vi "FA25_FW_pendulum_L3_4_0.vi"() -> ()   [LabVIEW 2025]
uses:
  <vilib>/Analysis/3filter.llb/Filter Passband Type.ctl
  Lab 3/FA25_pend_Lab3_4/SADI_Pendulum_lib/pendulumApp.lvlib
  <vilib>/ptbypt/NI_PtbyPt.lvlib
  <vilib>/Analysis/NI_AALBase.lvlib
panel:
  out "command":dbl
  in  "Tab Control":T1(tab)=enum."Plant and Controller"
  out "Firmware Version":sgl=1.002
  out "Software Version":dbl=1.104 format="%_6g"
  out "Number of SADI":i32=1
  out "reset":i32
  out "SADI Connect":i32
  out "P query":i32
  out "P start":i32
  in  "Desired DAQ Loop \nTime (ms)":dbl=0.2
  out "Actual DAQ Loop \nTime (ms)":dbl=0.20860000000084256 format="%#_7g"
  out "Elapsed \nTime (s) daq loop":dbl=15.046546899999953
  out "Txlat_ms":dbl=1.778
  out "min Txlat":dbl=0.682 format="%0.6f"
  out "max TXlat":dbl=4.932 format="%0.6f"
  out "std dev TXlat":dbl=0.7050052541669608 format="%0.6f"
  out "mean  TXlat":dbl=1.2022235999999924 format="%0.6f"
  out "Tx latency, ms":T2(graph)={"X Values"=[0.70325, 0.74575, 0.7882500000000001, 0.8307500000000001, 0.8732500000000001, 0.9157500000000001, 0.95825, 1.00075, 1.04325, 1.0857500000000002, 1.1282500000000002, 1.1707500000000002, 1.2132500000000002, 1.2557500000000001, 1.2982500000000001, 1.34075, 1.38325, 1.42575, 1.46825, 1.51075, 1.55325, 1.59575, 1.63825, 1.68075, 1.72325, 1.76575, 1.8082500000000004, 1.8507500000000003, 1.8932500000000003, 1.9357500000000003, 1.9782500000000003, 2.02075, 2.06325, 2.10575, 2.14825, 2.19075, 2.23325, 2.27575, 2.31825, 2.36075, 2.40325, 2.44575, 2.48825, 2.53075, 2.57325, 2.61575, 2.65825, 2.7007499999999998, 2.7432499999999997, 2.7857499999999997, 2.8282499999999997, 2.8707499999999997, 2.9132499999999997, 2.95575, 2.99825, 3.04075, 3.08325, 3.12575, 3.16825, 3.21075, 3.25325, 3.29575, 3.33825, 3.38075, 3.42325, 3.46575, 3.50825, 3.55075, 3.59325, 3.63575, 3.67825, 3.72075, 3.7632499999999998, 3.8057499999999997, 3.84825, 3.89075, 3.93325, 3.97575, 4.01825, 4.0607500000000005, 4.10325, 4.1457500000000005, 4.18825, 4.2307500000000005, 4.27325, 4.31575, 4.35825, 4.40075, 4.44325, 4.48575, 4.52825, 4.57075, 4.61325, 4.65575, 4.698250000000001, 4.74075, 4.783250000000001, 4.82575, 4.868250000000001, 4.91075], "Histogram: h(x)"=[155, 338, 552, 840, 858, 795, 153, 0, 0, 0, 0, 0, 0, 0, 0, 0, 0, 0, 0, 0, 0, 0, 0, 5, 49, 156, 220, 199, 196, 149, 0, 0, 0, 0, 0, 0, 0, 0, 0, 0, 0, 0, 0, 0, 0, 0, 0, 17, 26, 34, 37, 44, 58, 6, 0, 0, 0, 0, 0, 0, 0, 0, 0, 0, 0, 0, 0, 0, 0, 0, 0, 5, 5, 19, 5, 41, 7, 0, 0, 0, 0, 0, 0, 0, 0, 0, 0, 0, 0, 0, 0, 0, 0, 0, 0, 4, 0, 3, 0, 24]}
  out "ENC VEL":dbl=0.5175486320891765
  out "Pend Rot Error":dbl
  out "Pend Rot Filt":dbl=nan format="%0.2f"
  out "Pendulum velocity":dbl=3.5305560095629e-285
  out "Platen velocity":dbl=0.01738392532814515
  out "Command":dbl=-14.479572053947942
  out "desired\nposition":dbl=-14.790379679306856
  out "Platen Rot Error":dbl format="%0.2f"
  in  "Frequency":dbl=0.5
  in  "Amplitude":dbl=100.0
  in  "Turn On Command":dbl=40.0
  in  "Stop":bool=TRUE
  in  "Desired Loop \nTime (ms)":dbl=1.0
  out "Actual Loop Time (ms)":dbl=1.0000979999995252
  out "Elapsed Time (s)":dbl=15.048252700000035
  out "Segments Saved":u32
  in  "Save Data?":bool
  out "ENC POS":i32=-761
  out "Pendulum ENC":i32
  in  "Sine/Square":bool=TRUE
  in  "Enable Motor":bool=TRUE
  in  "Output Units":enum16{"Degrees", "Radians"}(ring)
  in  "Couts/rev":dbl=3704.0
  in  "Zero":bool
  out "Platen Rotation":dbl=-73.96328293736501
  out "Command Graph":T3(graph)={"Desired Rotation/Command"=-14.479572053947942, -14.479572053947942, 0.0, 0.0}
  out "Desired vs Actual Platen Angle Graph":cluster{"sine wave":dbl, "Filtered x":dbl}(graph)={"sine wave"=-14.479572053947942, "Filtered x"=-73.96328293736501}
  out "Pendulum Rotation Graph":cluster{dbl, dbl}(graph)={nan, 0.0}
  in  "n-int":i32=100
  in  "n-diff":i32=5
  in  "Sampling freq: fs":dbl=1000.0
  in  "Cutoff freq: fl":dbl=10.0 format="%0.3f"
  in  "initialize":bool
  out "PendEncValMax":u16=3687
  out "PendEncValMin":u16=3178
  in  "Pendulum Zero":bool
  out "Pend Rotation":dbl=1440.0 format="%0.2f"
  in  "k1":dbl
  in  "k2":dbl
  in  "k3":dbl
  in  "k4":dbl
  out "u":dbl
  in  "k5":dbl
  out "Read Call Error Out":u16(ring)=32768 items=["SADI_RESET (FT_OK)"=0, "FT_INVALID_HANDLE"=1, "FT_DEVICE_NOT_FOUND"=2, "FT_DEVICE_NOT_OPENED"=3, "FT_IO_ERROR"=4, "FT_INSUFFICIENT_RESOURCES"=5, "FT_OTHER_ERROR"=18, "FT_NOT_SUPPORTED"=17, "DATA_RECEIVED"=32768, "NO_DATA_AVAIL"=32769, "NO_SADI"=32770]
  out "SADI State":T4(ring)=enum."Close"
  # "Platen Rotation & Velocity"
  # "Signal Generator"
  # "Butterworth Filter Settings"
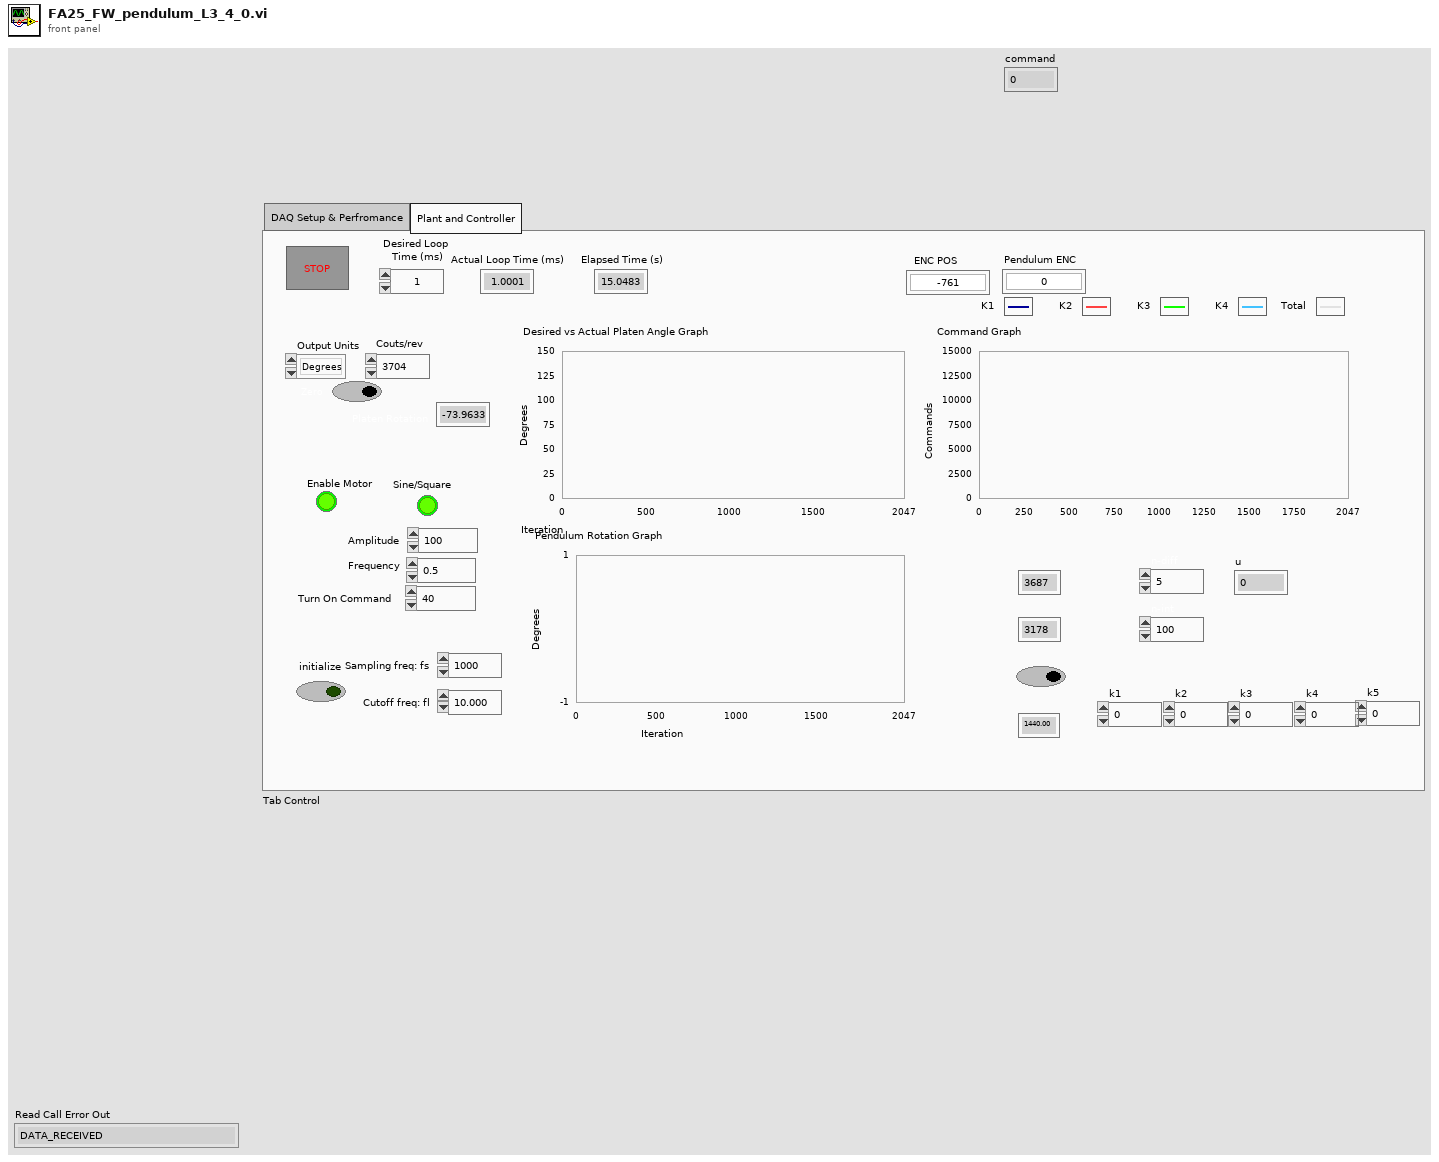
[diagram p1: front panel]
types:
  T1 = enum32{"DAQ Setup & Perfromance", "Plant and Controller"}
  T2 = cluster{"X Values":dbl[], "Histogram: h(x)":i32[]}
  T3 = cluster{"Desired Rotation/Command":dbl, dbl, dbl, dbl}
  T4 = enum32{"SADI_check", "Connect_boot", "Check_SW_FW", "Pend_Start", "Run", "Stop", "Store", "Close"}
  T5 = typedef "NI_AALBase.lvlib/Filter Passband Type.ctl" = enum32{"Lowpass", "Highpass", "Bandpass", "Bandstop"}
  T6 = cluster{"desired\nposition":dbl, "Platen Rotation":dbl}
  T7 = cluster{"desired\nposition":dbl, "Command":dbl, dbl, dbl}
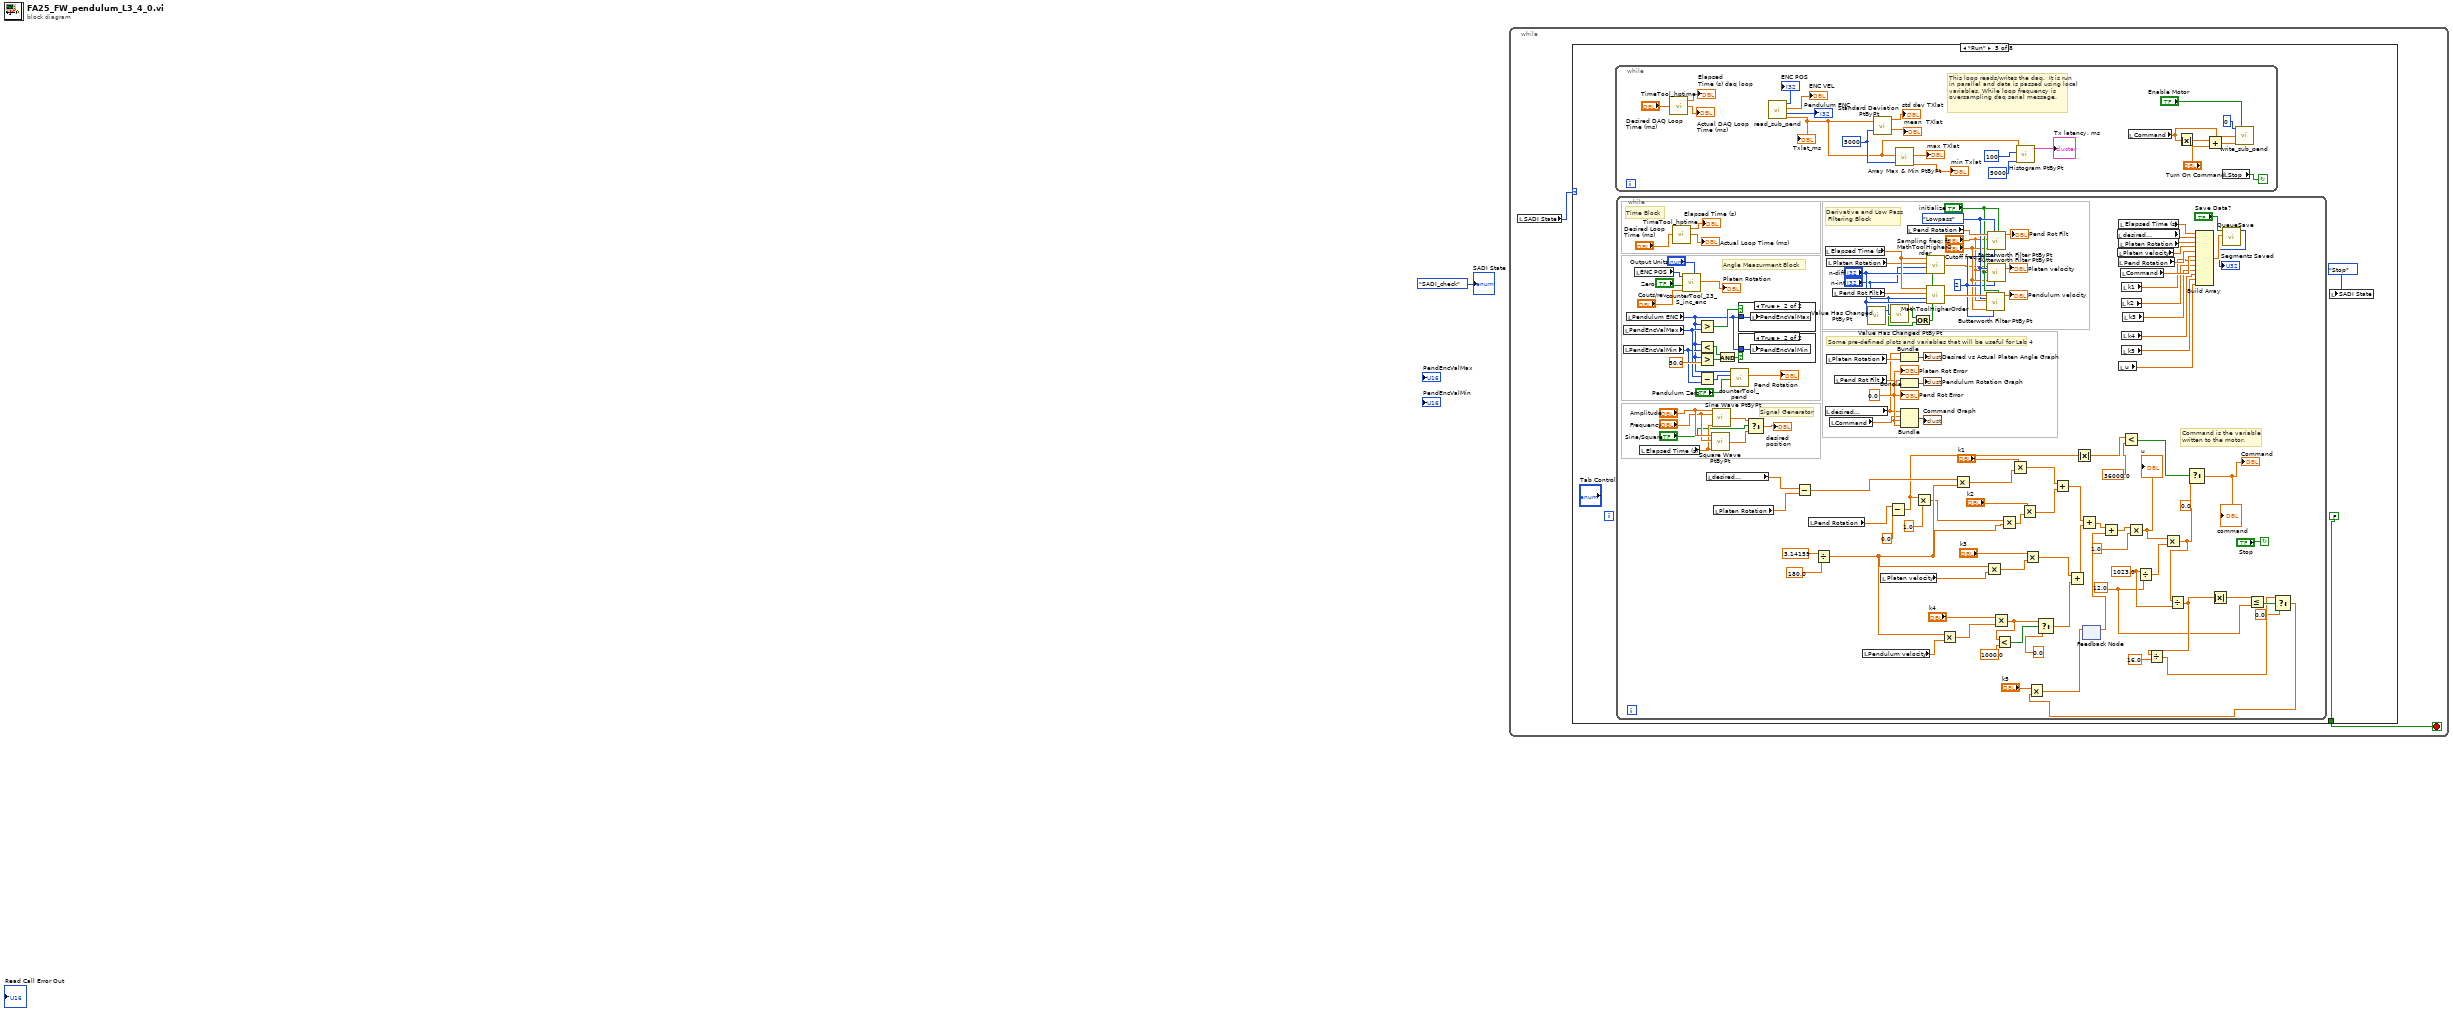
[diagram p0: block diagram]
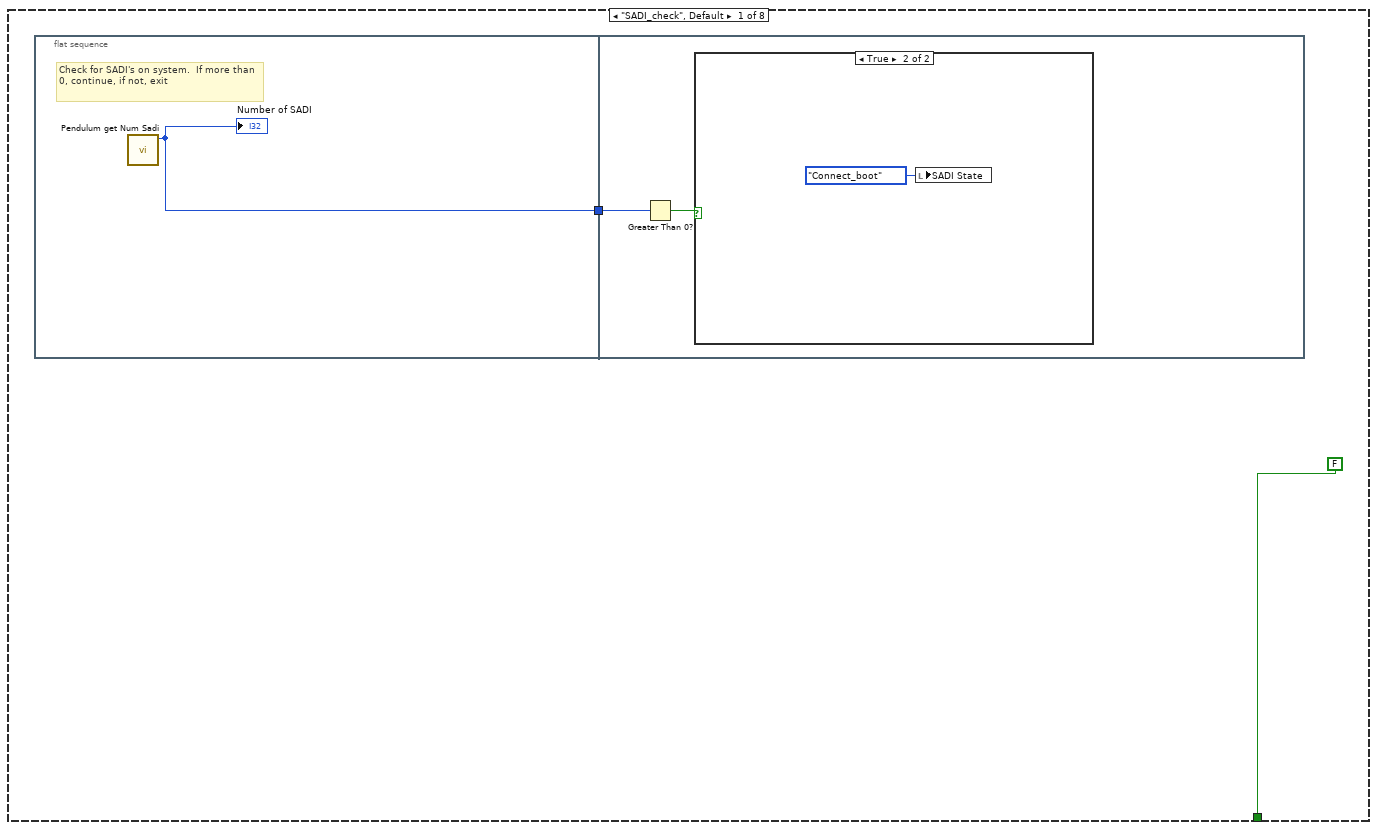
[diagram p2: hidden frame]
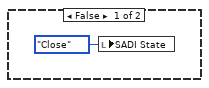
[diagram p3: hidden frame]
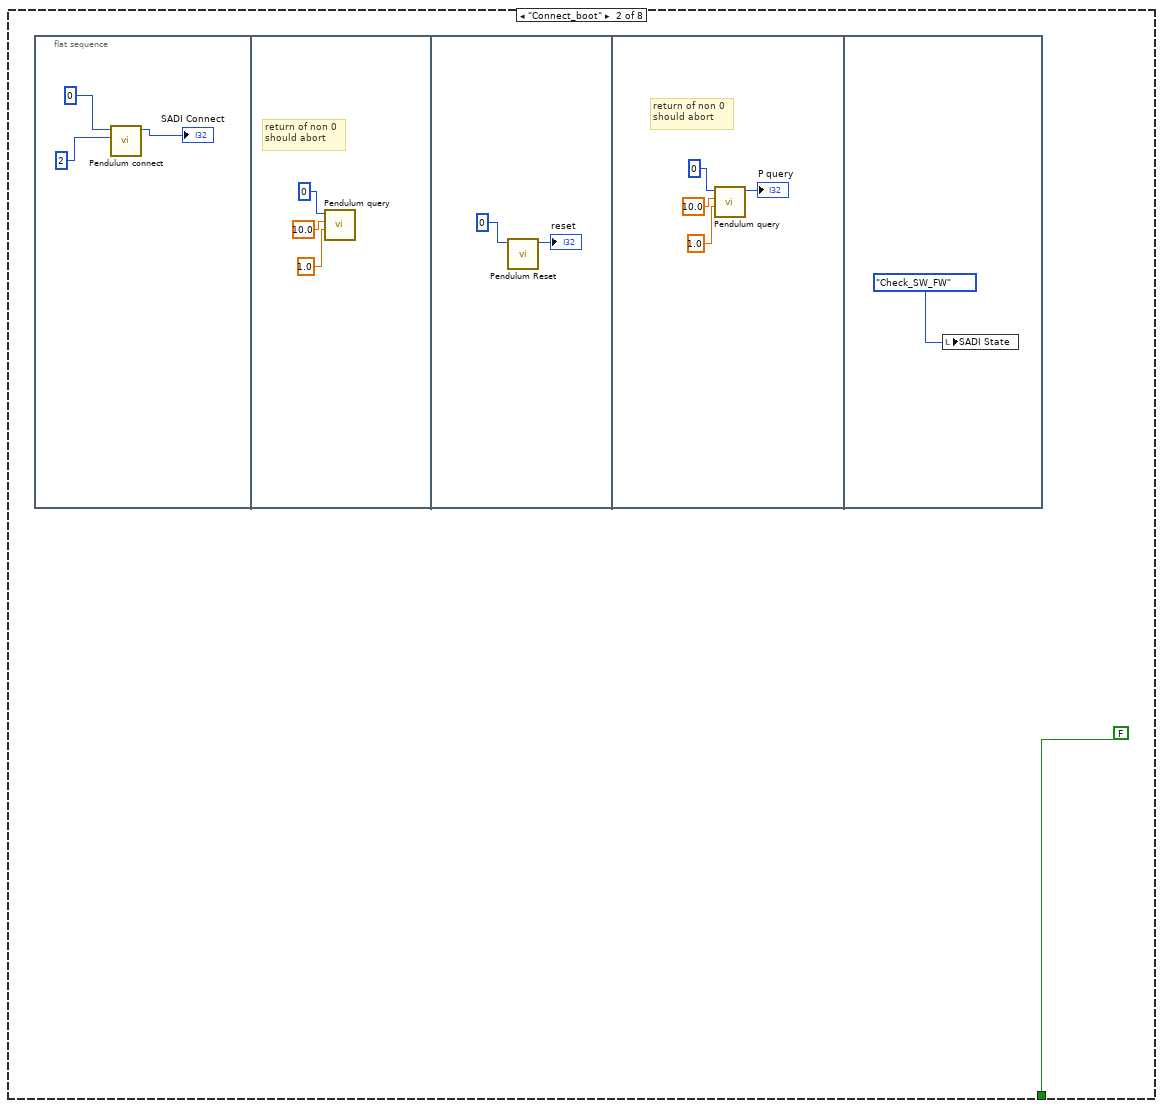
[diagram p4: hidden frame]
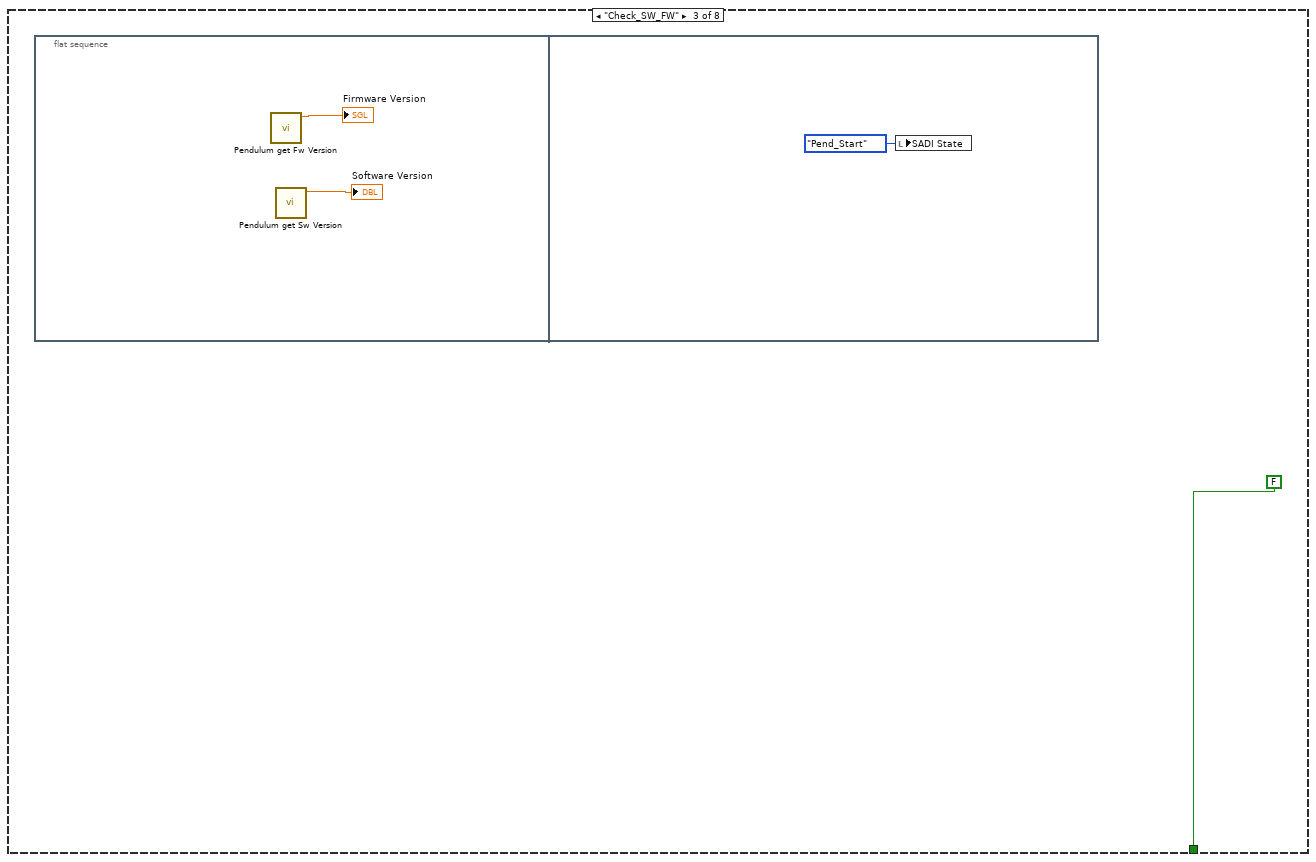
[diagram p5: hidden frame]
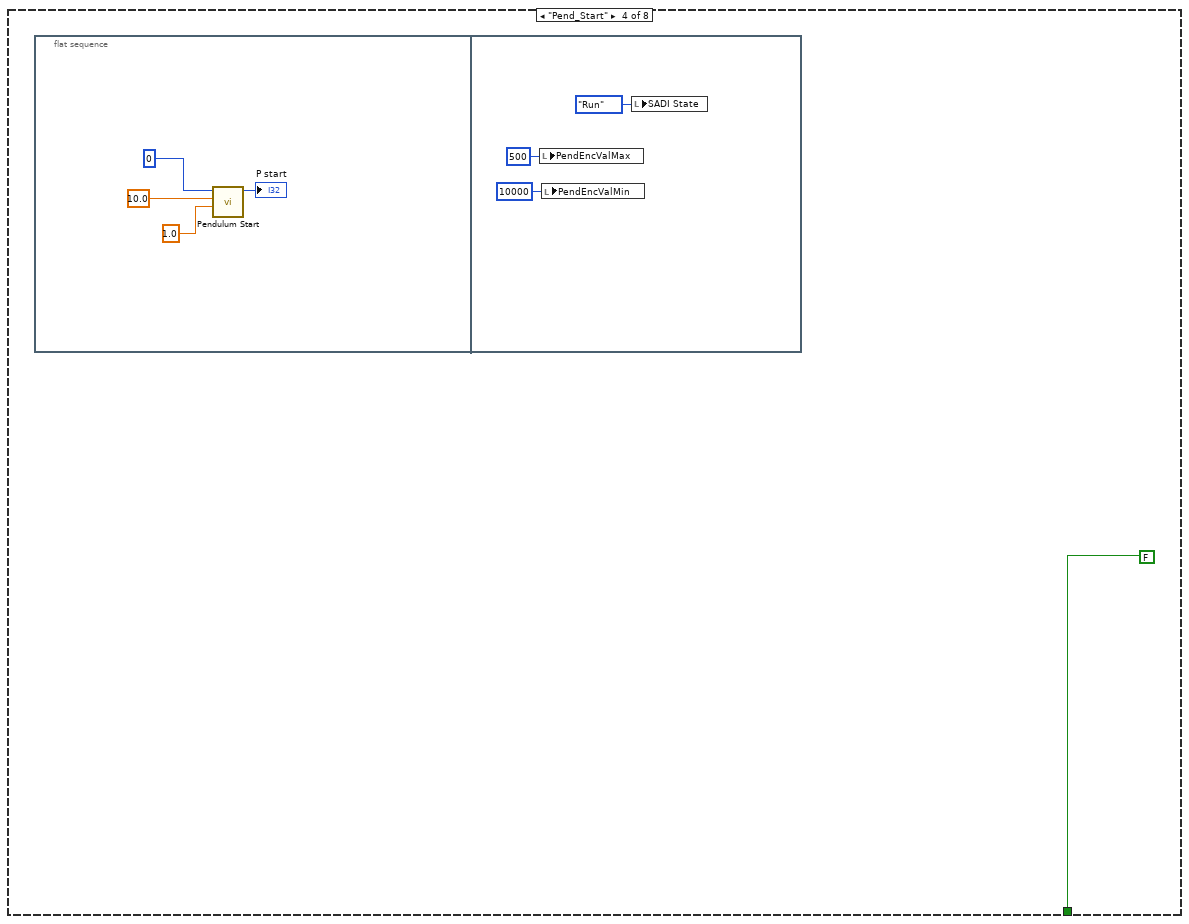
[diagram p6: hidden frame]
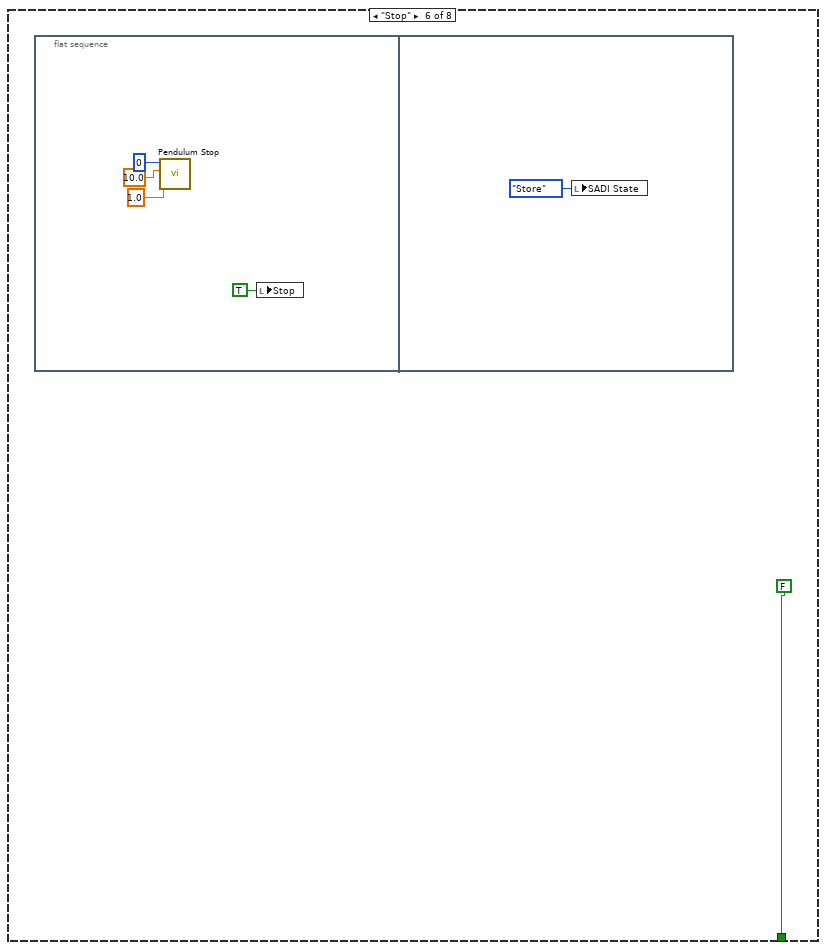
[diagram p9: hidden frame]
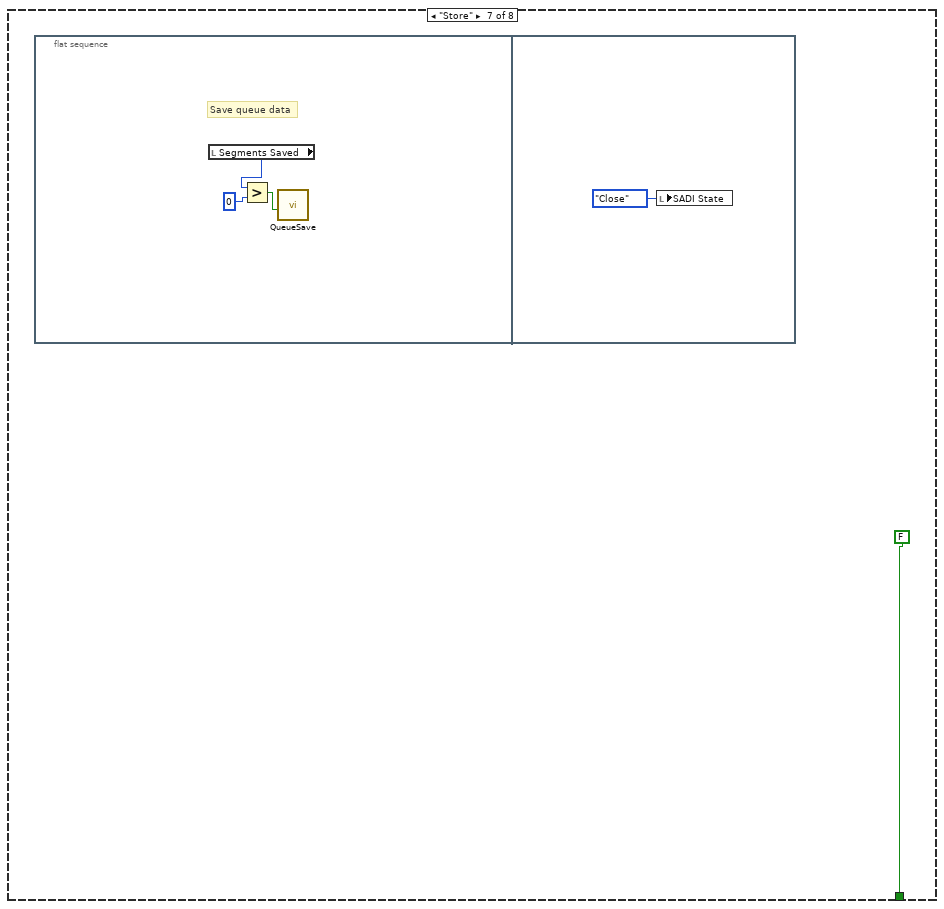
[diagram p10: hidden frame]
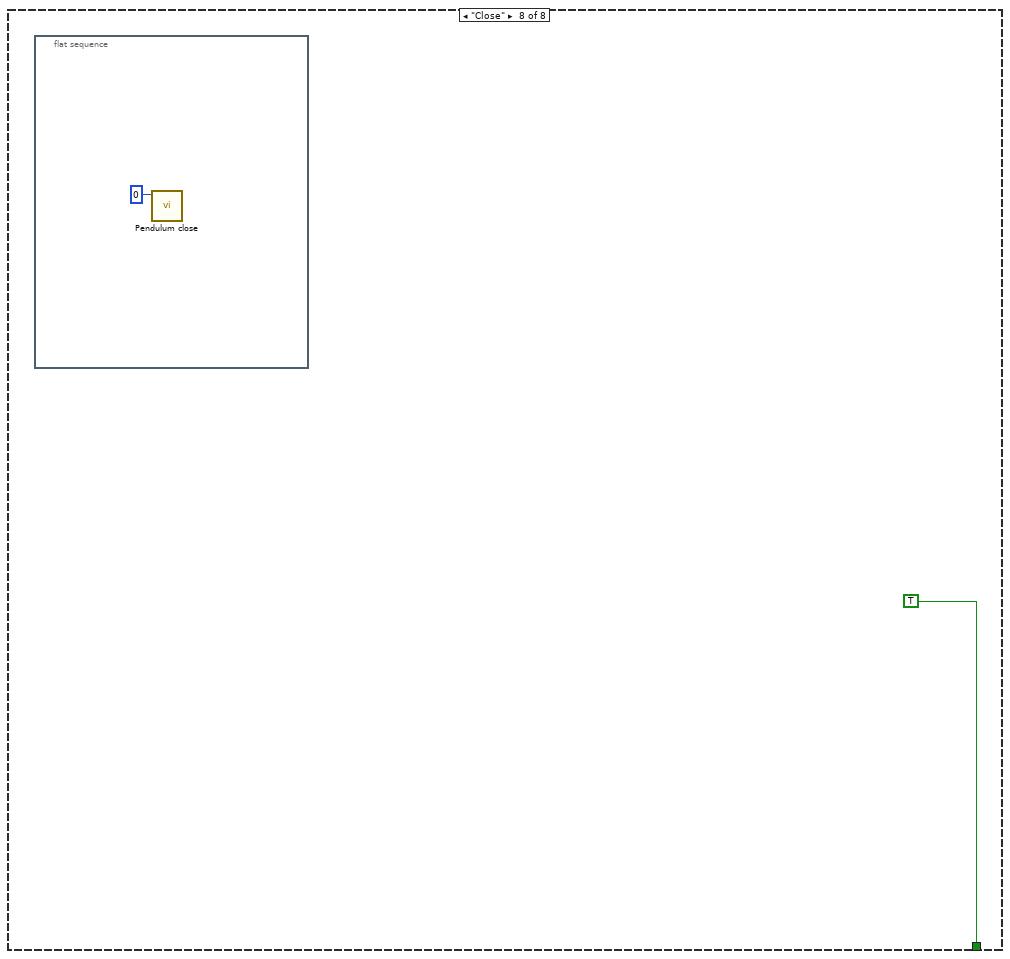
[diagram p11: hidden frame]
diagram:
  n1 = while {
    stop <- w2 stop-if-true
    n2 = local read "SADI State"() -> (w3:T4)
    n3 = case shown="\"Run\"" w3 {
      tunnel: [FALSE FALSE FALSE FALSE FALSE FALSE FALSE TRUE] -> w2
      frame "SADI_check", Default {
        n4 = flat-sequence {
          tunnel: [w6] -> w5
          tunnel: w5 -> [w7]
          frame #0 {
            # "Check for SADI's on system.  If more than 0, continue, if not, exit"
            n5 = call "Pendulum get Num Sadi.vi"() -> ("function return"=w6:i32)  [unwired: 11 in]
            "Number of SADI" <- w6
          }
          frame #1 {
            n6 = Greater Than 0?(x=w7) -> (x > 0?=w8:bool)
            n7 = case shown="True" w8 {
              frame False {
                n8 = local write "SADI State"(T4."Close" ("SADI State")) -> ()
              }
              frame True {
                n9 = local write "SADI State"(T4."Connect_boot" ("SADI State")) -> ()
              }
            }
          }
        }
      }
      frame "Connect_boot" {
        n10 = flat-sequence {
          frame #0 {
            n11 = call "Pendulum connect.vi"("latency_mS"=u8 2, "instance"=0) -> ("function return"=→"SADI Connect":i32)  [unwired: 9 in]
          }
          frame #1 {
            # "return of non 0\nshould abort"
            n12 = call "Pendulum query.vi"("timeout_sec"=1.0, "retry_ms"=10.0, "instance"=0) -> ()  [unwired: 8 in, 1 out]
          }
          frame #2 {
            n13 = call "Pendulum Reset.vi"("instance"=0) -> ("function return"=→"reset":i32)  [unwired: 10 in]
          }
          frame #3 {
            # "return of non 0\nshould abort"
            n14 = call "Pendulum query.vi"("timeout_sec"=1.0, "retry_ms"=10.0, "instance"=0) -> ("function return"=→"P query":i32)  [unwired: 8 in]
          }
          frame #4 {
            n15 = local write "SADI State"(T4."Check_SW_FW" ("SADI State")) -> ()
          }
        }
      }
      frame "Check_SW_FW" {
        n16 = flat-sequence {
          frame #0 {
            n17 = call "Pendulum get Fw Version.vi"() -> ("function return"=→"Firmware Version":dbl)  [unwired: 11 in]
            n18 = call "Pendulum get Sw Version.vi"() -> ("function return"=→"Software Version":dbl)  [unwired: 11 in]
          }
          frame #1 {
            n19 = local write "SADI State"(T4."Pend_Start" ("SADI State")) -> ()
          }
        }
      }
      frame "Pend_Start" {
        n20 = flat-sequence {
          frame #0 {
            n21 = call "Pendulum Start.vi"("timeout_sec"=1.0, "retry_mS"=10.0, "instance"=0) -> ("function return"=→"P start":i32)  [unwired: 8 in]
          }
          frame #1 {
            n22 = local write "PendEncValMax"(u16 500 ("PendEncValMax")) -> ()
            n23 = local write "PendEncValMin"(u16 10000 ("PendEncValMin")) -> ()
            n24 = local write "SADI State"(T4."Run" ("SADI State")) -> ()
          }
        }
      }
      frame "Run" {
        n25 = while {
          stop <- w40 continue-if-true
          w54 = 5000 ("sample length")
          # "This loop reads/writes the daq.  It is run in parallel and data is passed using local variables. While loop frequency is oversampling daq serial message."
          n26 = call "TimeTool_hptime.vi"("Desired Loop Time (ms)"="Desired DAQ Loop \nTime (ms)") -> ("elapsed time (s)"=→"Elapsed \nTime (s) daq loop":dbl, "dt (ms)"=→"Actual DAQ Loop \nTime (ms)":dbl)  [unwired: 1 out]
          n27 = call "read_sub_pend.vi"() -> ("Txlat_ms"=w49:dbl, "Pendulum ENC 2"=→"Pendulum ENC":i32, "ENC VEL 1"=→"ENC VEL":dbl, "ENC POS 1"=→"ENC POS":i32)  [unwired: 7 in]
          "Txlat_ms" <- w49
          n28 = call <vilib>:"Standard Deviation PtByPt.vi"("x"=w49, "sample length"=w54) -> ("standard deviation"=→"std dev TXlat":dbl, "mean"=→"mean  TXlat":dbl)  [unwired: 1 in, 1 out]
          n29 = call <vilib>:"Array Max & Min PtByPt.vi"("input data point"=w49, "sample length"=w54) -> ("max value"=→"max TXlat":dbl, "min value"=→"min Txlat":dbl)  [unwired: 1 in, 3 out]
          n30 = call <vilib>:"Histogram PtByPt.vi"("sample length"=5000, "intervals"=100, "x"=w49) -> ("Histogram Graph"=→"Tx latency, ms":T2)  [unwired: 5 in, 3 out]
          n31 = local read "Command"() -> (w39:dbl)
          n32 = Absolute Value(x=w39) -> (abs(x)=w45:dbl)
          n33 = Add(x=w45, y="Turn On Command") -> (x+y=w46:dbl)
          n34 = local read "Stop"() -> (w40:bool)
          n35 = call "write_sub_pend.vi"("instance"=0, "Enable Motor"="Enable Motor", "direction"=w39, "motorEffort"=w46) -> ()  [unwired: 12 in]
        }
        n36 = while {
          stop <- "Stop" continue-if-true
          w80 = 12.0 ("y")
          w89 = 1023.0 ("x")
          w129 = 0.0
          w139 = 2 ("order")
          w141 = Filter_Passband_Type."Lowpass" ("filter type")
          # "Command is the variable \nwritten to the motor."
          # "Some pre-defined plots and variables that will be useful for Lab 4"
          # "Derivative and Low Pass\n FIltering Block"
          # "Angle Measurment Block"
          # "Signal Generator"
          # "Time Block"
          n37 = local read "PendEncValMax"() -> (w155:u16)
          n38 = local read "PendEncValMin"() -> (w154:u16)
          n39 = local read "Pendulum ENC"() -> (w152:i32)
          n40 = local read "ENC POS"() -> (w166:i32)
          n41 = local read "Elapsed Time (s)"() -> (w174:dbl)
          n42 = call "TimeTool_hptime.vi"("Desired Loop Time (ms)"="Desired Loop \nTime (ms)") -> ("elapsed time (s)"=→"Elapsed Time (s)":dbl, "dt (ms)"=→"Actual Loop Time (ms)":dbl)  [unwired: 1 out]
          n43 = call "counterTool_23_S_inc_enc.vi"("Counts"=w166, "Zero"="Zero", "Couts/rev"="Couts/rev", "Output Units"="Output Units") -> ("Total Angle"=→"Platen Rotation":dbl)  [unwired: 3 in, 1 out]
          n44 = Greater?(x=w152, y=w155) -> (0:w159:bool)
          n45 = Less?(x=w152, y=w154) -> (x < y?=w161:bool)
          n46 = Greater?(x=w152, y=50.0) -> (0:w160:bool)
          n47 = Subtract(x=w155, y=w154) -> (x-y=w156:u16)
          n48 = local read "desired\nposition"() -> (w74:dbl)
          n49 = call <vilib>:"Square Wave PtByPt.vi"("amplitude"="Amplitude", "frequency"="Frequency", "time"=w174) -> ("square wave"=w171:dbl)  [unwired: 2 in]
          n50 = call <vilib>:"Sine Wave PtByPt.vi"("time"=w174, "frequency"="Frequency", "amplitude"="Amplitude") -> ("sine wave"=w172:dbl)  [unwired: 1 in]
          n51 = local read "Platen Rotation"() -> (w75:dbl)
          n52 = And(x=w161, y=w160) -> (x .and. y?=w158:bool)
          n53 = call "counterTool_pend.vi"("Counts"=w152, "Pendulum Scale"=w156, "Zero"="Pendulum Zero") -> ("Total Angle"=→"Pend Rotation":dbl)  [unwired: 4 in, 1 out]
          n54 = case shown="True" w159 {
            tunnel: w152 -> [_ w185]
            frame False {
            }
            frame True {
              n55 = local write "PendEncValMax"(w185) -> ()
            }
          }
          n56 = case shown="True" w158 {
            tunnel: w152 -> [_ w184]
            frame False {
            }
            frame True {
              n57 = local write "PendEncValMin"(w184) -> ()
            }
          }
          n58 = Select(t=w172, s="Sine/Square", f=w171) -> (s? t:f=→"desired\nposition":dbl)
          n59 = Subtract(x=w74, y=w75) -> (x-y=w73:dbl)
          n60 = local read "Pend Rotation"() -> (w72:dbl)
          n61 = Divide(x=3.14159, y=180.0) -> (x/y=w98:dbl)
          n62 = local read "Elapsed Time (s)"() -> (w150:dbl)
          n63 = local read "desired\nposition"() -> (w122:dbl)
          n64 = local read "Platen Rotation"() -> (w128:dbl)
          n65 = local read "Platen Rotation"() -> (w145:dbl)
          n66 = local read "Command"() -> (w121:dbl)
          n67 = local read "Pend Rot Filt"() -> (w144:dbl)
          n68 = local read "Pend Rot Filt"() -> (w127:dbl)
          n69 = local read "Pendulum velocity"() -> (w99:dbl)
          n70 = call <vilib>:"Value Has Changed PtByPt.vi"("input data point"="n-diff") -> ("has changed"=w133:bool)  [unwired: 1 in, 1 out]
          n71 = local read "Platen velocity"() -> (w102:dbl)
          n72 = Subtract(x=w72, y=0.0) -> (x-y=w70:dbl)
          n73 = call <vilib>:"Value Has Changed PtByPt.vi"("input data point"="n-int") -> ("has changed"=w134:bool)  [unwired: 1 in, 1 out]
          n74 = Bundle("desired\nposition"=w122, "Platen Rotation"=w128) -> (→"Desired vs Actual Platen Angle Graph":T6)  [unwired: 1 in]
          n75 = Bundle("Pend Rot Filt"=w127, w129) -> (→"Pendulum Rotation Graph":cluster{"Pend Rot Filt":dbl, dbl})  [unwired: 1 in]
          n76 = Bundle("desired\nposition"=w122, "Command"=w121, w129, w129) -> (→"Command Graph":T7)  [unwired: 1 in]
          n77 = local read "Pend Rotation"() -> (w146:dbl)
          n78 = Or(x=w134, y=w133) -> (x .or. y?=w148:bool)
          n79 = Multiply(x=w70, y=1.0) -> (x*y=w69:dbl)
          n80 = call "MathToolHigherOrder.vi"("Time"=w150, "Data"=w145, "n-int"="n-int", "Reset (F)"=w148, "n-diff"="n-diff") -> ("1st derivative"=w135:dbl)  [unwired: 1 in, 2 out]
          n81 = call "MathToolHigherOrder.vi"("Time"=w150, "Data"=w144, "n-int"="n-int", "Reset (F)"=w148, "n-diff"="n-diff") -> ("1st derivative"=w142:dbl)  [unwired: 1 in, 2 out]
          n82 = Multiply(x=w98, y=w99) -> (x*y=w100:dbl)
          n83 = Multiply(x=w73, y=w98) -> (x*y=w109:dbl)
          n84 = Multiply(x=w98, y=w102) -> (x*y=w101:dbl)
          n85 = call <vilib>:"Butterworth Filter PtByPt.vi"("initialize"="initialize", "order"=w139, "filter type"=w141, "low cutoff freq: fl"="Cutoff freq: fl", "sampling freq: fs"="Sampling freq: fs", "x"=w142) -> ("Filtered x"=→"Pendulum velocity":dbl)  [unwired: 3 in, 1 out]
          n86 = call <vilib>:"Butterworth Filter PtByPt.vi"("initialize"="initialize", "order"=w139, "filter type"=w141, "low cutoff freq: fl"="Cutoff freq: fl", "sampling freq: fs"="Sampling freq: fs", "x"=w146) -> ("Filtered x"=→"Pend Rot Filt":dbl)  [unwired: 3 in, 1 out]
          n87 = call <vilib>:"Butterworth Filter PtByPt.vi"("initialize"="initialize", "order"=w139, "filter type"=w141, "low cutoff freq: fl"="Cutoff freq: fl", "sampling freq: fs"="Sampling freq: fs", "x"=w135) -> ("Filtered x"=→"Platen velocity":dbl)  [unwired: 3 in, 1 out]
          n88 = Multiply(x="k4", y=w100) -> (x*y=w106:dbl)
          n89 = Less?(x=w106, y=1000.0) -> (x < y?=w104:bool)
          n90 = Multiply(x=w69, y=w98) -> (x*y=w97:dbl)
          n91 = Multiply(x="k1", y=w109) -> (x*y=w116:dbl)
          n92 = Multiply(x="k2", y=w97) -> (x*y=w115:dbl)
          n93 = Multiply(x="k3", y=w101) -> (x*y=w114:dbl)
          n94 = Select(t=w106, s=w104, f=0.0) -> (s? t:f=w103:dbl)
          n95 = Add(x=w116, y=w115) -> (x+y=w113:dbl)
          n96 = Add(x=w114, y=w103) -> (x+y=w112:dbl)
          n97 = Absolute Value(x=w70) -> (abs(x)=w94:dbl)
          n98 = Add(x=w113, y=w112) -> (x+y=w85:dbl)
          n99 = feedback #1() -> (w83:dbl)  [unwired: 1 in]
          n100 = Add(x=w85, y=w83) -> (x+y=w86:dbl)
          n101 = local read "desired\nposition"() -> (w163:dbl)
          n102 = local read "Platen velocity"() -> (w125:dbl)
          n103 = local read "Pend Rotation"() -> (w124:dbl)
          n104 = local read "Elapsed Time (s)"() -> (w182:dbl)
          n105 = local read "Platen Rotation"() -> (w126:dbl)
          n106 = local read "u"() -> (w62:dbl)
          n107 = local read "Command"() -> (w123:dbl)
          n108 = local read "k2"() -> (w66:dbl)
          n109 = local read "k1"() -> (w67:dbl)
          n110 = local read "k4"() -> (w64:dbl)
          n111 = local read "k5"() -> (w63:dbl)
          n112 = Less?(x=w94, y=36000.0) -> (x < y?=w92:bool)
          n113 = local read "k3"() -> (w65:dbl)
          n114 = Multiply(x=w86, y=1.0) -> (x*y=w111:dbl)
          "u" <- w111
          n115 = Divide(x=w89, y=w80) -> (x/y=w110:dbl)
          n116 = Multiply(x=w111, y=w110) -> (x*y=w90:dbl)
          n117 = Divide(x=w90, y=w89) -> (x/y=w82:dbl)
          n118 = Divide(x=w82, y=16.0) -> (x/y=w78:dbl)
          n119 = Select(t=w90, s=w92, f=0.0) -> (s? t:f=→"Command" →"command":dbl)
          n120 = Build Array(w182, w163, w126, w125, w124, w123, w67, w66, w65, w64, w63, w62) -> (w181:dbl[])
          n121 = Absolute Value(x=w82) -> (abs(x)=w81:dbl)
          n122 = call "QueueSave.vi"("Data In"=w181, "Save Data?"="Save Data?") -> ("Segments Saved"=→"Segments Saved":u32)  [unwired: 3 in, 2 out]
          n123 = Less Or Equal?(x=w81, y=w80) -> (x <= y?=w79:bool)
          n124 = Select(t=w78, s=w79, f=0.0) -> (s? t:f=w77:dbl)
          n125 = Multiply(x="k5", y=w77) -> (x*y=w84:dbl)
          n126 = feedback-in #1(w84) -> ()
          "Platen Rot Error" <- w129
          "Pend Rot Error" <- w129
        }
        n127 = local write "SADI State"(T4."Stop" ("SADI State")) -> ()
      }
      frame "Stop" {
        n128 = flat-sequence {
          frame #0 {
            n129 = call "Pendulum Stop.vi"("timeout_sec"=1.0, "retry_mS"=10.0, "instance"=0) -> ()  [unwired: 8 in, 1 out]
            n130 = local write "Stop"(TRUE ("Stop")) -> ()
          }
          frame #1 {
            n131 = local write "SADI State"(T4."Store" ("SADI State")) -> ()
          }
        }
      }
      frame "Store" {
        n132 = flat-sequence {
          frame #0 {
            # "Save queue data"
            n133 = local read "Segments Saved"() -> (w195:u32)
            n134 = Greater?(x=w195, y=u32 0) -> (0:w194:bool)
            n135 = call "QueueSave.vi"("Write To Spreadsheet"=w194) -> ()  [unwired: 4 in, 3 out]
          }
          frame #1 {
            n136 = local write "SADI State"(T4."Close" ("SADI State")) -> ()
          }
        }
      }
      frame "Close" {
        n137 = flat-sequence {
          frame #0 {
            n138 = call "Pendulum close.vi"("instance"=0) -> ()  [unwired: 10 in, 1 out]
          }
        }
      }
    }
  }
  "SADI State" <- T4."SADI_check" ("SADI State")
